vi "REF add remove phase element.vi"(1 "NewVal in":T1={"Ch"=[13.0], " f (Hz)"=[], "Phase (°)"=[], "TC (s)"=[0.0], "order"=[0.0]} {"order" format="%#_3g"; "TC (s)" format="%#_3p"; "Phase (°)" format="%#_3g"}) -> (0 "NewVal out":T1={"Ch"=[13.0], " f (Hz)"=[], "Phase (°)"=[], "TC (s)"=[0.0], "order"=[0.0]} {"order" format="%#_3g"; "TC (s)" format="%#_3p"; "Phase (°)" format="%#_3g"})   [LabVIEW 2016, in "Instrument.Lockin.lvclass"]
uses:
  Instrument.Lockin.lvclass
  LockinDAQ/Typedefs/REF-cluster.ctl
  LockinDAQ/LockinDAQ.lvclass
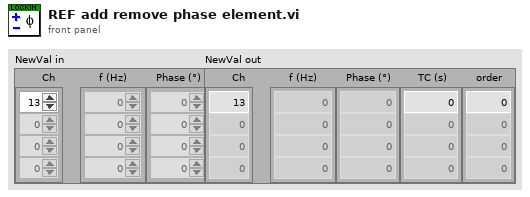
[diagram p1: front panel]
types:
  T1 = typedef "LockinDAQ.lvclass/REF-cluster.ctl" = cluster{"Ch":dbl[], " f (Hz)":dbl[], "Phase (°)":dbl[], "TC (s)":dbl[], "order":dbl[]}
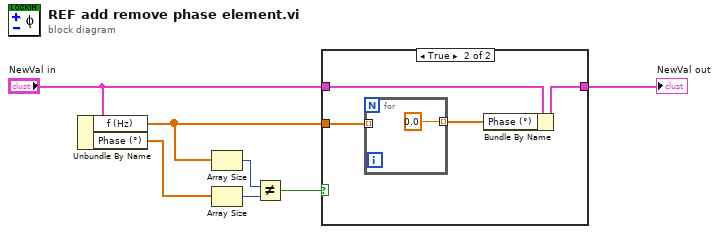
[diagram p0: block diagram]
diagram:
  n1 = Unbundle By Name("NewVal in") -> ("f (Hz)"=w6:dbl[], "Phase (°)"=w5:dbl[])
  n2 = Array Size(array=w6) -> (size(s)=w4:i32)
  n3 = Array Size(array=w5) -> (size(s)=w7:i32)
  n4 = Not Equal?(x=w4, y=w7) -> (x != y?=w3:bool)
  n5 = case shown="True" w3 {
    tunnel: w6 -> [_ w12]
    tunnel: "NewVal in" -> [w8 w10]
    tunnel: [w8 w9] -> w1
    frame False {
    }
    frame True {
      n6 = for {
        tunnel: w12 -> [_] mode=indexing
        tunnel: [0.0] -> w11 mode=indexing
      }
      n7 = Bundle By Name(cluster=w10, "Phase (°)"=w11) -> (w9:T1)
    }
  }
  "NewVal out" <- w1
